vi "FileDialog.vi"(8 "error in":errorcluster, 11 "start path":path=path "") -> (0 "error out":errorcluster, 1 "cancelled":bool, 3 "selected path":path)   [LabVIEW 2015, in "Configuration Tool.lvlib"]
doc: "Opens a Dialog for getting the file Path for the configurationCopyright 2017 National Instruments Corporation\n\nLicensed under the Apache License, Version 2.0 (the \"License\"); you may not use this file except in compliance with the License. You may obtain a copy of the License at http://www.apache.org/licenses/LICENSE-2.0\nUnless required by applicable law or agreed to in writing, software distributed under the License is distributed on an \"AS IS\" BASIS, WITHOUT WARRANTIES OR CONDITIONS OF ANY KIND, either express or implied. See the License for the specific language governing permissions and limitations under the License."
uses:
  Configuration Tool.lvlib
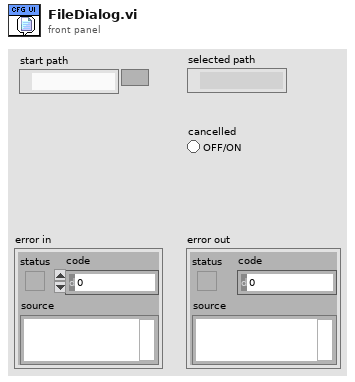
[diagram p1: front panel]
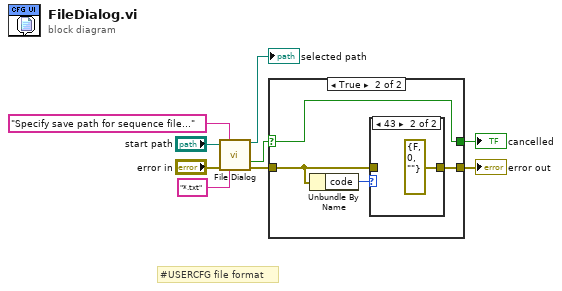
[diagram p0: block diagram]
diagram:
  # "#USERCFG file format"
  n1 = call "File Dialog"("start path"="start path", "prompt"="Specify save path for sequence file..." ("Prompt"), "error in"="error in", "pattern (all files)"="*.txt" ("pattern")) -> ("selected path"=→"selected path":path, "cancelled"=w8:bool, "error out"=w9:errorcluster)  [unwired: 8 in, 1 out]
  n2 = case shown="True" w8 {
    selector: w8 -> [w10 w12]
    tunnel: w9 -> [w11 w14]
    tunnel: [w11 w13] -> w6
    tunnel: [w10 w12] -> w7
    frame False {
    }
    frame True {
      n3 = Unbundle By Name(w14) -> ("code"=w15:i32)
      n4 = case shown="43" w15 {
        tunnel: w14 -> [w16 _]
        tunnel: [w16 errorcluster {"status"=FALSE, "code"=0, "source"=""} ("error out")] -> w13
        frame Default {
        }
        frame 43 {
        }
      }
    }
  }
  "cancelled" <- w7
  "error out" <- w6
